vi "Launch New Build.vi"(6 "Build Number":string, 7 "Automated Rebuild":bool, 8 "error in (no error)":errorcluster, 9 "Name of target (My Computer)":string="My Computer", 10 "Name of build specification (if empty: build all)":string, 11 "Path to project":path) -> (0 "error out":errorcluster)   [LabVIEW 2018]
uses:
  <vilib>/AppBuilder/AB_API_Simple/Build (path).vi
  <vilib>/AppBuilder/AB_API_Simple/NI_App_Builder_API.lvlib
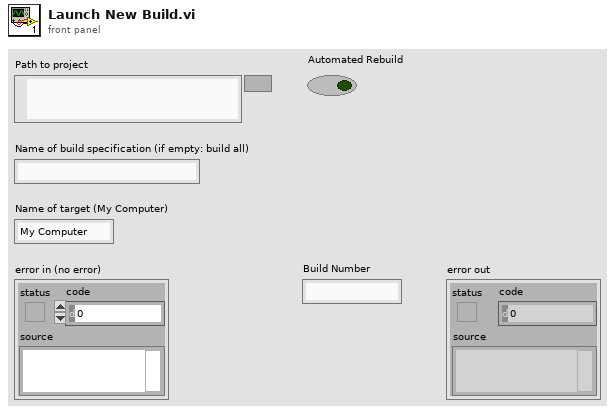
[diagram p1: front panel]
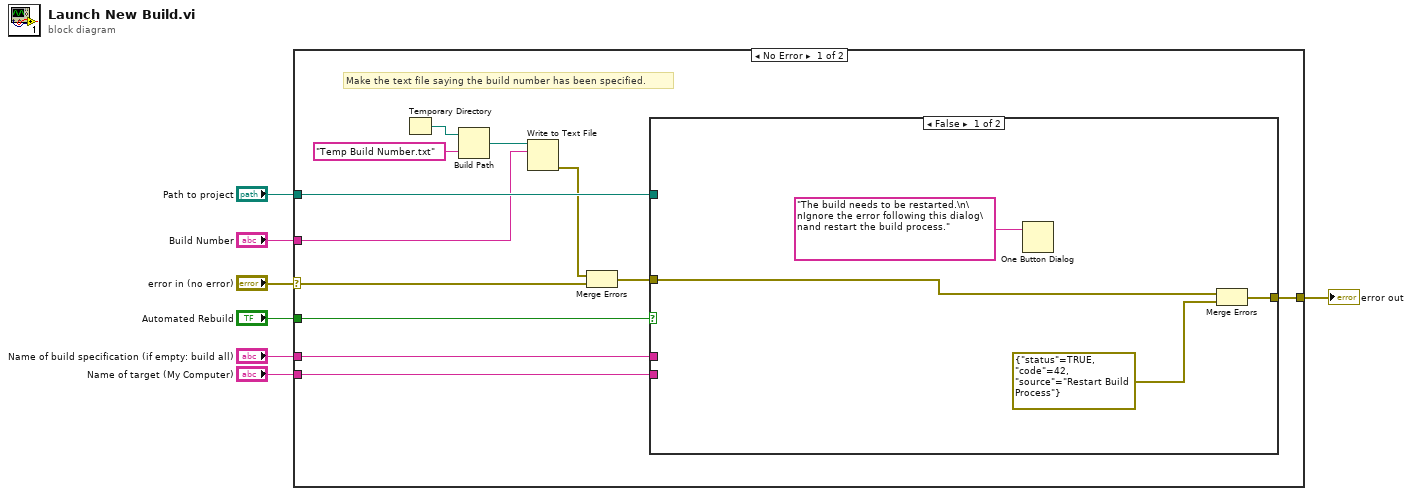
[diagram p0: block diagram]
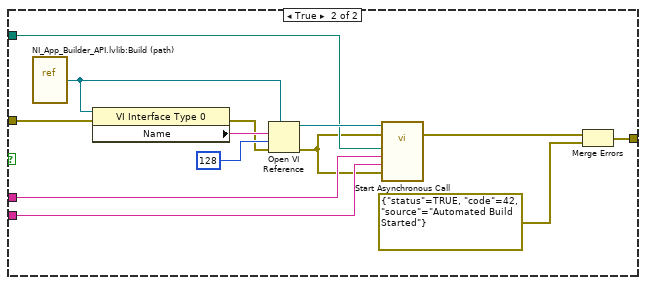
[diagram p2: hidden frame]
diagram:
  n1 = case shown="No Error" "error in (no error)" {
    selector: "error in (no error)" -> [w16 w37]
    tunnel: "Path to project" -> [w19 _]
    tunnel: "Name of build specification (if empty: build all)" -> [w18 _]
    tunnel: "Name of target (My Computer)" -> [w17 _]
    tunnel: [w15 w37] -> w3
    tunnel: "Build Number" -> [w11 _]
    tunnel: "Automated Rebuild" -> [w8 _]
    frame No Error {
      # "Make the text file saying the build number has been specified."
      n2 = Temporary Directory() -> (w14:path)
      n3 = Build Path(base path=w14, name or relative path="Temp Build Number.txt") -> (appended path=w12:path)
      n4 = Write to Text File(file (use dialog)=w12, text=w11) -> (error out=w9:errorcluster)  [unwired: 2 in, 2 out]
      n5 = Merge Errors(w9, w16) -> (w10:errorcluster)
      n6 = case shown="False" w8 {
        tunnel: w19 -> [_ w32]
        tunnel: w18 -> [_ w31]
        tunnel: w17 -> [_ w30]
        tunnel: [w21 w24] -> w15
        tunnel: w10 -> [w22 w27]
        frame False {
          n7 = One Button Dialog(message="The build needs to be restarted.\n\nIgnore the error following this dialog\nand restart the build process.") -> ()  [unwired: 1 in, 1 out]
          n8 = Merge Errors(w22, errorcluster {"status"=TRUE, "code"=42, "source"="Restart Build Process"} ("error IO")) -> (w21:errorcluster)
        }
        frame True {
          n9 = vi-ref "NI_App_Builder_API.lvlib:Build (path).vi"() -> (w36:refnum<vi>)
          n10 = property class="VI Interface Type 0"(reference=w36, error in=w27) -> (error out=w29:errorcluster, "Name"=w35:string)  [unwired: 1 out]
          n11 = Open VI Reference(type specifier VI Refnum (for type only)=w36, vi path=w35, options=128, error in (no error)=w29) -> (vi reference=w33:refnum<vi>, error out=w28:errorcluster)  [unwired: 2 in]
          n12 = call-by-ref "Start Asynchronous Call"(reference=w33, error in=w28, 8:"error in (no error)"=w28, "Name of target (My Computer)"=w30, "Name of build specification (if empty: build all)"=w31, "Path to project"=w32) -> (error out=w25:errorcluster)  [unwired: 6 in, 3 out]
          n13 = Merge Errors(w25, errorcluster {"status"=TRUE, "code"=42, "source"="Automated Build Started"} ("error IO")) -> (w24:errorcluster)
        }
      }
    }
    frame Error {
    }
  }
  "error out" <- w3
